vi "Reason_Select.vi"(8 "error in (no error)":errorcluster, 11 "Ref in":T1={"MS SQL Connection"=refnum, "UDL File"=path "", "Time"="", "DCODE"="", "WIP+1"=0, "MC No?"=0, "POKAYOKE?"=FALSE, "Expected Result"="", "Result [Status]"="", "Clock"=0.0, "RFID"="", "WIP Queue"=refnum, "TS Parameter"={"ProfitCenterCode"="", "LineCode"="", "WorkOrderNumber"="", "Model"="", "Model_with_Prefix"="", "VendorCode"="", "SetParameterDateCode"="", "PokaYoke"=0, "Target"=1, "Live_DateCode"="", "CustomerPartNumber"="", "Hand"="", "sBarcode"=FALSE, "FCA"=0, "Ent_Stamp"=timestamp(0 s since 1904-01-01), "STS_CD"=0.0}, "Data_Queue"=[], "RFID Serial No."=""} {"TS Parameter"."FCA" format="%01d"; "TS Parameter"."Target" min=1 max=100000; "TS Parameter"."PokaYoke" min=0 max=1}) -> (0 "error out":errorcluster, 2 "Cancel?":bool, 3 "Reason Out":string)   [LabVIEW 2020]
uses:
  Controls/TD SQL.ctl
  <vilib>/addons/database/Connection.llb/Conn ObjectReference.ctl
  Controls/WIP_State.ctl
  Controls/TS_Parameter.ctl
  <vilib>/addons/database/Connection.llb/Conn Execute.vi
  <vilib>/addons/database/NI_Database_API.lvlib
panel:
  in  "Select":bool
  in  "Cancel":bool
  in  "Reason":string
  in  "Reason List":u16(ring) items=["Barcode Mismatch", "Barcode Missing"]
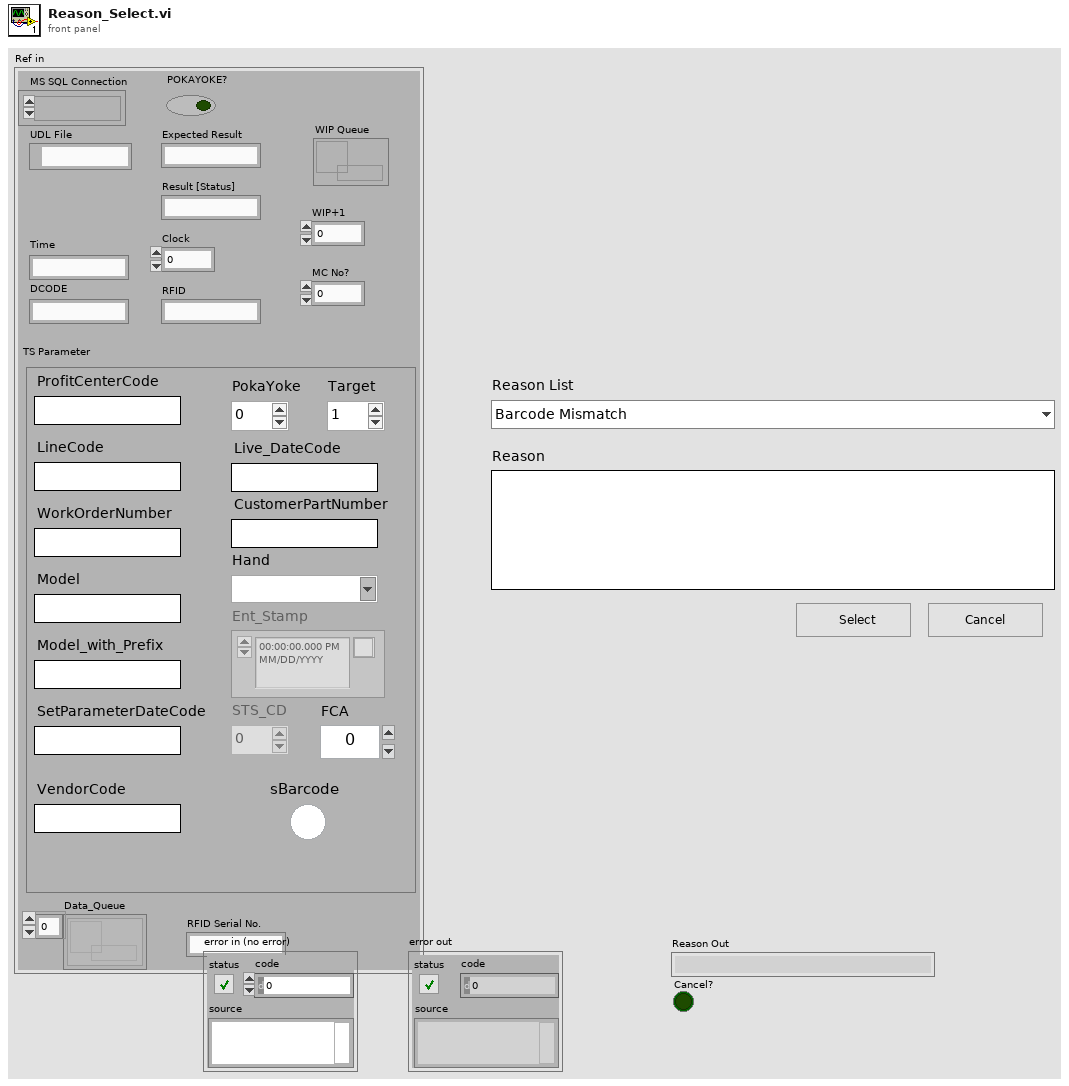
[diagram p1: front panel]
types:
  T1 = typedef "TD SQL.ctl" = cluster{"MS SQL Connection":T2, "UDL File":path, "Time":string, "DCODE":string, "WIP+1":i64, "MC No?":i32, "POKAYOKE?":bool, "Expected Result":string, "Result [Status]":string, "Clock":dbl, "RFID":string, "WIP Queue":refnum<queue>, "TS Parameter":T3, "Data_Queue":refnum<queue>[], "RFID Serial No.":string}
  T2 = typedef "NI_Database_API.lvlib/Conn ObjectReference.ctl" = refnum<k1>
  T3 = typedef "TS_Parameter.ctl" = cluster{"ProfitCenterCode":string, "LineCode":string, "WorkOrderNumber":string, "Model":string, "Model_with_Prefix":string, "VendorCode":string, "SetParameterDateCode":string, "PokaYoke":i32, "Target":i32, "Live_DateCode":string, "CustomerPartNumber":string, "Hand":string, "sBarcode":bool, "FCA":i32, "Ent_Stamp":timestamp, "STS_CD":dbl}
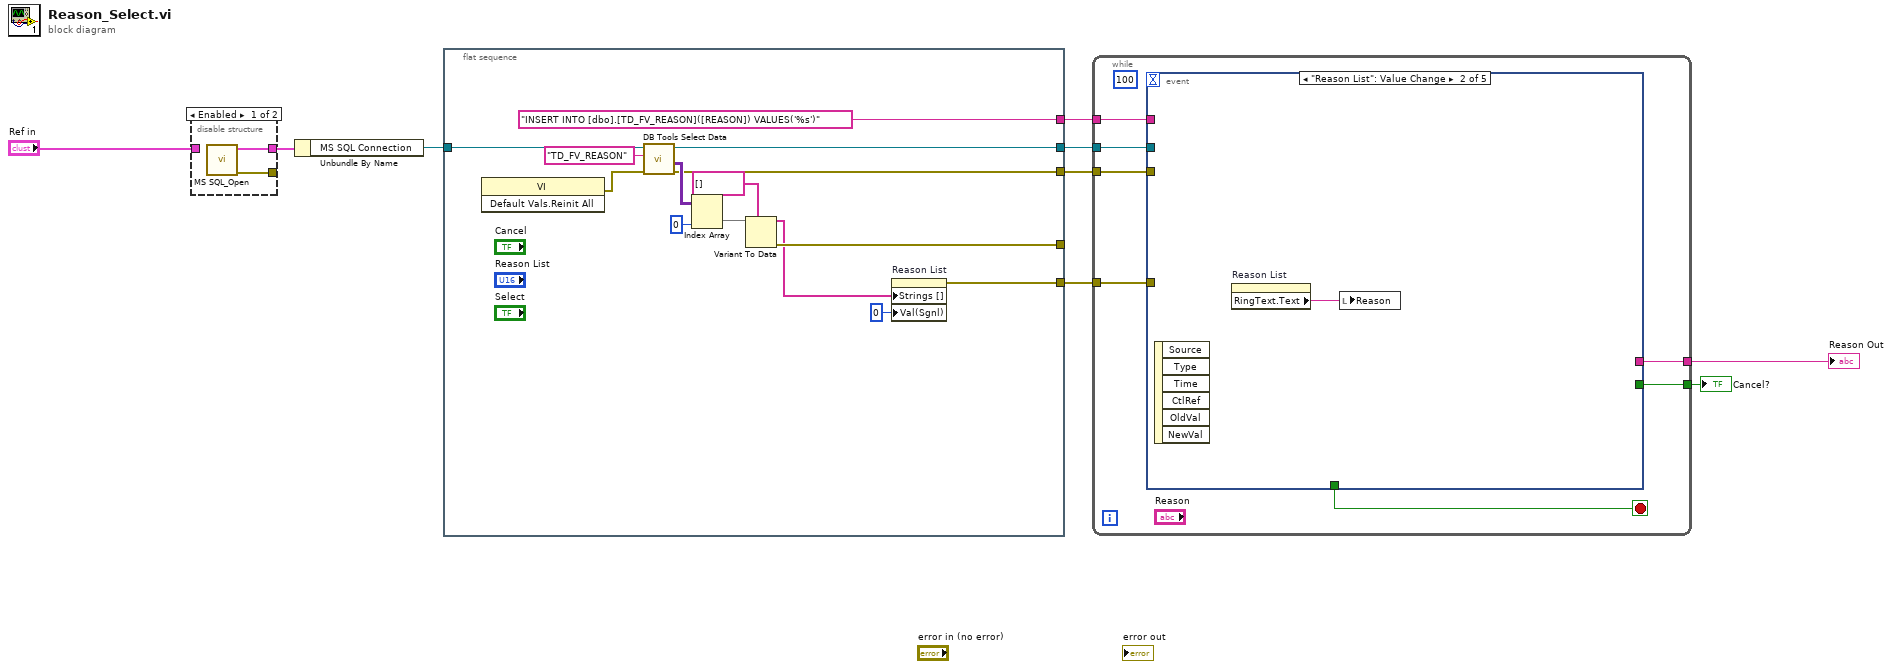
[diagram p0: block diagram]
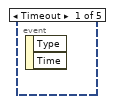
[diagram p2: hidden frame]
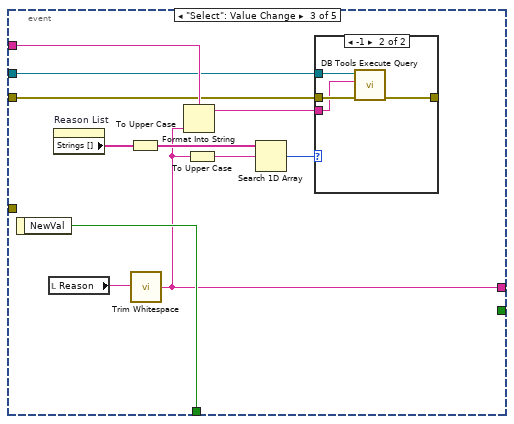
[diagram p3: hidden frame]
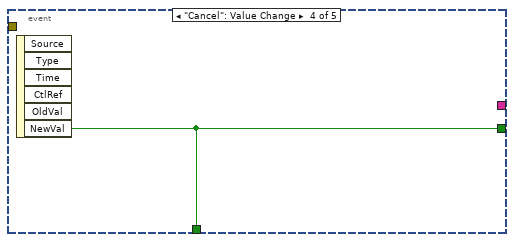
[diagram p5: hidden frame]
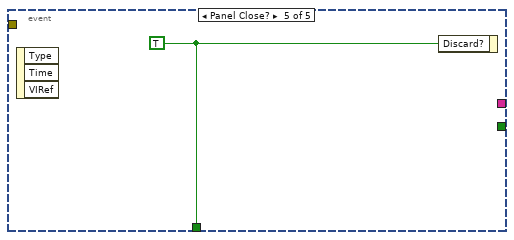
[diagram p6: hidden frame]
diagram:
  n1 = disable-structure shown="Enabled" {
    disable-tunnel: [w11 w12] -> w9
    disable-tunnel: "Ref in" -> [_ w12]
    disable-tunnel: [w10 _] -> _
    frame Enabled {
      n2 = call "MS SQL_Open.vi"() -> ("error out"=w10:errorcluster, "Ref Out"=w11:T1)  [unwired: 9 in, 1 out]
    }
    frame Disabled {
    }
  }
  n3 = Unbundle By Name(w9) -> ("MS SQL Connection"=w7:T2)
  n4 = flat-sequence {
    tunnel: w7 -> [w26]
    tunnel: [w20] -> w4
    tunnel: [w19] -> _
    tunnel: [w16] -> w6
    tunnel: [w14] -> w5
    tunnel: ["INSERT INTO [dbo].[TD_FV_REASON]([REASON]) VALUES('%s')" ("String")] -> w2
    frame #0 {
      n5 = invoke class="VI" method="Default Vals.Reinit All"() -> (error out=w15:errorcluster)  [unwired: 3 in, 2 out]
      n6 = call <vilib>:"DB Tools Select Data.vi"("error in (no error)"=w15, "table"="TD_FV_REASON", "connection reference"=w26) -> ("error out"=w20:errorcluster, "data"=w24:variant[][], "connection reference out"=w14:T2)  [unwired: 3 in]
      n7 = Index Array(array=w24, index (col)=0 ("disabled index (col)")) -> (element=w22:variant[])  [unwired: 1 in]
      n8 = Variant To Data(type=string[] [] ("columns"), Variant=w22) -> (data=w18:string[], error out=w19:errorcluster)  [unwired: 1 in]
      n9 = property on="Reason List" class="Ring (strict)"("Strings []"=w18, "Val(Sgnl)"=u16 0 ("Value (Signaling)")) -> (error out=w16:errorcluster)  [unwired: 2 in, 1 out]
    }
  }
  n10 = while {
    tunnel: w6 -> [w32]
    tunnel: w5 -> [w31]
    tunnel: w4 -> [w30]
    tunnel: [w29] -> w3
    tunnel: w2 -> [w28]
    tunnel: [w27] -> w1
    stop <- w33 stop-if-true
    (unwired) 100
    n11 = event shown="[1] \"Reason List\": Value Change" {
      selector: _ -> [_ _ _ _ _]
      dyn-events: _ -> [_ _ _ _ _]
      timeout: _ -> [_ _ _ _ _]
      tunnel: [_ _ w45 w50 w51] -> w33
      tunnel: w32 -> [_ _ _ _ _]
      tunnel: w31 -> [_ _ w38 _ _]
      tunnel: w30 -> [_ _ w37 _ _]
      tunnel: [_ _ w39 _ _] -> w29
      tunnel: w28 -> [_ _ w40 _ _]
      tunnel: [_ _ _ w50 _] -> w27
      event Timeout {
        n12 = event-data() -> ()  [unwired: 1 in, 2 out]
      }
      event "Reason List": Value Change {
        n13 = event-data() -> ()  [unwired: 1 in, 6 out]
        n14 = property on="Reason List" class="Ring (strict)"() -> ("RingText.Text"=w34:string)  [unwired: 2 in, 2 out]
        n15 = local write "Reason"(w34) -> ()
      }
      event "Select": Value Change {
        n16 = event-data() -> ("NewVal"=w45:bool)  [unwired: 1 in]
        n17 = local read "Reason"() -> (w35:string)
        n18 = property on="Reason List" class="Ring (strict)"() -> ("Strings []"=w44:string[])  [unwired: 2 in, 2 out]
        n19 = To Upper Case(1:w44) -> (0:w43:string[])
        n20 = call <vilib>:"Trim Whitespace.vi"("string"=w35) -> ("trimmed string"=w39:string)  [unwired: 1 in]
        n21 = Format Into String(format string=w40, w39) -> (resulting string=w36:string)  [unwired: 2 in, 1 out]
        n22 = To Upper Case(1:w39) -> (0:w42:string)
        n23 = Search 1D Array(1D array=w43, element=w42) -> (index of element=w41:i32)  [unwired: 1 in]
        n24 = case shown="-1" w41 {
          tunnel: w38 -> [_ w49]
          tunnel: w37 -> [_ w48]
          tunnel: w36 -> [_ w47]
          tunnel: [_ w46] -> _
          frame 0, Default {
          }
          frame -1 {
            n25 = call-poly <vilib>:"DB Tools Execute Query.vi"("error in (no error)"=w48, "SQL query"=w47, "connection reference"=w49) -> ("error out"=w46:errorcluster)  [unwired: 5 in, 1 out]
          }
        }
      }
      event "Cancel": Value Change {
        n26 = event-data() -> ("NewVal"=w50:bool)  [unwired: 1 in, 5 out]
      }
      event Panel Close? {
        w51 = TRUE ("Discard?")
        n27 = event-data() -> ()  [unwired: 1 in, 3 out]
        n28 = event-data("Discard?"=w51) -> ()  [unwired: 1 in, 1 out]
      }
    }
  }
  "Reason Out" <- w3
  "Cancel?" <- w1
